vi "update Norm.vi"(8 "error in (no error)":errorcluster, 10 "Norm.lvclass":refnum<class "Norm.lvclass">, 11 "Report in":refnum<class "Report.lvclass">) -> (0 "error out":errorcluster, 3 "Report out":refnum<class "Report.lvclass">)   [LabVIEW 2013, in "DatenKlassen.lvlib" / "Report.lvclass"]
uses:
  Report.lvclass
  Norm/Norm.lvclass
  Report.lvclass/Report.ctl
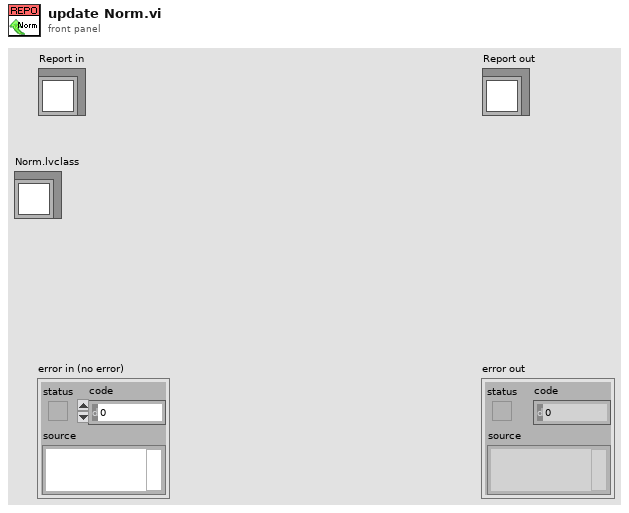
[diagram p1: front panel]
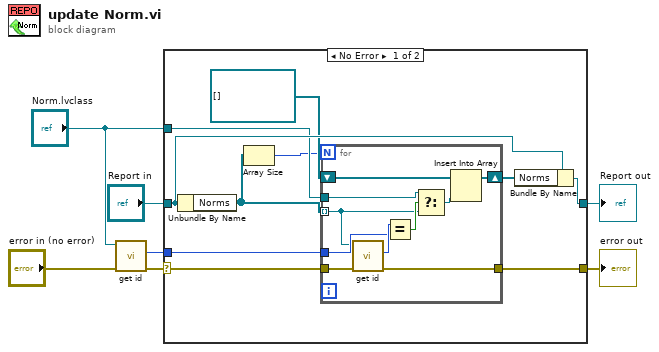
[diagram p0: block diagram]
diagram:
  n1 = call-dynamic "get id.vi"("error in (no error)"="error in (no error)", "Norm (Eingang)"="Norm.lvclass") -> ("error out"=w1:errorcluster, "id"=w3:i32)  [unwired: 7 in, 1 out]
  n2 = case shown="No Error" w1 {
    selector: w1 -> [w17 w29]
    tunnel: [w13 w29] -> w7
    tunnel: [w14 w28] -> w5
    tunnel: "Report in" -> [w15 w28]
    tunnel: w3 -> [w16 _]
    tunnel: "Norm.lvclass" -> [w12 _]
    frame No Error {
      n3 = Unbundle By Name(w15) -> ("Norms"=w9:refnum<class "Norm.lvclass">[])
      n4 = Array Size(array=w9) -> (size(s)=w8:i32)
      n5 = for {
        N: w8 -> [_]
        tunnel: w9 -> [w21] mode=indexing
        tunnel: w17 -> [w27]
        tunnel: w16 -> [w25]
        tunnel: w12 -> [w22]
        tunnel: [w24] -> w13
        shift-right: [w18] -> w10
        shift-left: refnum<class "Norm.lvclass">[] [] ("Norms") -> [w20]
        n6 = call-dynamic "get id.vi"("error in (no error)"=w27, "Norm (Eingang)"=w21) -> ("error out"=w24:errorcluster, "id"=w26:i32)  [unwired: 7 in, 1 out]
        n7 = Equal?(x=w26, y=w25) -> (x = y?=w23:bool)
        n8 = Select(t=w22, s=w23, f=w21) -> (s? t:f=w19:refnum<class "Norm.lvclass">)
        n9 = Insert Into Array(array=w20, new element=w19) -> (w18:refnum<class "Norm.lvclass">[])  [unwired: 1 in]
      }
      n10 = Bundle By Name(cluster=w15, "Norms"=w10) -> (w14:refnum<class "Report.lvclass">)
    }
    frame Error {
    }
  }
  "error out" <- w7
  "Report out" <- w5
